vi "Get ReadWrite Data Refs.vi"(8 "error in (no error)":errorcluster, 10 "Hardware Output Refs":T1[](array[typedef]) format="%.0x", 11 "Device Ref":T1 format="%.0x") -> (0 "error out":errorcluster, 2 "Pairs":cluster{"Chan Refs":T2[], "Prev. Values":dbl[]} {"Chan Refs" format="%.0x"}, 3 "Device Ref out":T1=18446744073709551615 format="%.0x")   [LabVIEW 2015, in "Instrument Addon System Explorer.lvlib"]
uses:
  Instrument Addon System Explorer.lvlib
  <vilib>/NI Veristand/Custom Device API/Data Reference.ctl
  <vilib>/NI Veristand/Custom Device API/Custom Device Item Ref.ctl
  <vilib>/NI Veristand/Custom Device API/Data Access Type.ctl
  <vilib>/NI Veristand/Custom Device API/Custom Device API.lvlib
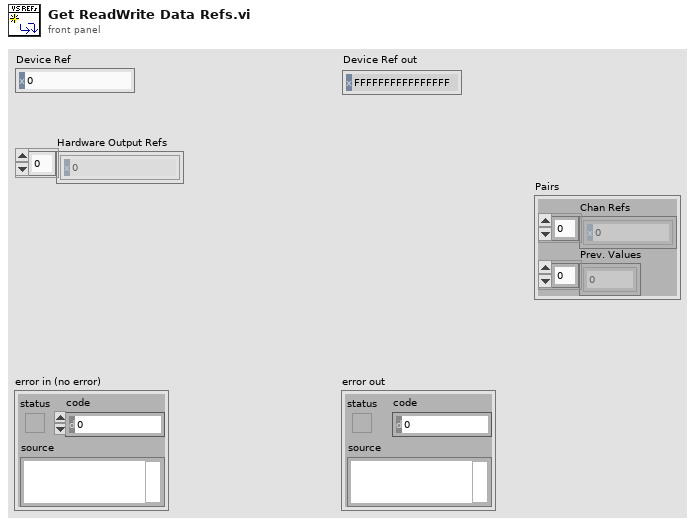
[diagram p1: front panel]
types:
  T1 = typedef "Custom Device API.lvlib/Custom Device Item Ref.ctl" = u64
  T2 = typedef "Custom Device API.lvlib/Data Reference.ctl" = i32
  T3 = typedef "Custom Device API.lvlib/Data Access Type.ctl" = enum16{"Read", "Write"}
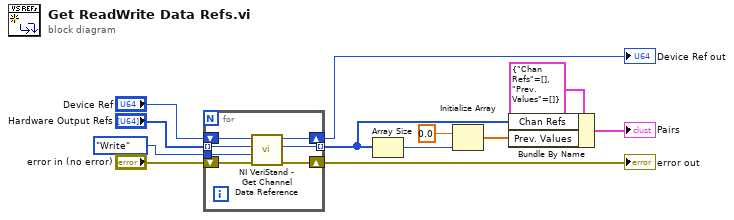
[diagram p0: block diagram]
diagram:
  n1 = for {
    tunnel: "Hardware Output Refs" -> [w15] mode=indexing
    tunnel: Data_Access_Type."Write" ("Access") -> [w14]
    shift-right: [w17] -> w4
    shift-left: "error in (no error)" -> [w18]
    shift-right: [w19] -> w3
    shift-left: "Device Ref" -> [w16]
    tunnel: [w13] -> w5 mode=indexing
    n2 = call <vilib>:"NI VeriStand - Get Channel Data Reference.vi"("error in (no error)"=w18, "Access"=w14, "Channel Ref in"=w15, "Device Ref in"=w16) -> ("error out"=w17:errorcluster, "Channel Data Reference"=w13:T2, "Device Ref out"=w19:T1)  [unwired: 5 in]
  }
  "error out" <- w4
  "Device Ref out" <- w3
  n3 = Array Size(array=w5) -> (size(s)=w7:i32)
  n4 = Initialize Array(0.0 ("element"), w7) -> (w6:dbl[])
  n5 = Bundle By Name(cluster=cluster{"Chan Refs":T2[], "Prev. Values":dbl[]} {"Chan Refs"=[], "Prev. Values"=[]} ("Pairs"), "Chan Refs"=w5, "Prev. Values"=w6) -> (→"Pairs":cluster{"Chan Refs":T2[], "Prev. Values":dbl[]})
